vi "Error站_Core.vi"(6 "Flag in":T1, 7 "Function":T6(ring)=enum."CloseReference", 8 "error in":errorcluster, 9 "Data in":T3, 10 "Name":string, 11 "ref in":T2) -> (0 "error out":errorcluster, 2 "Data out":T3, 3 "ref out":T2, 4 "Flag out":T1)   [LabVIEW 2015]
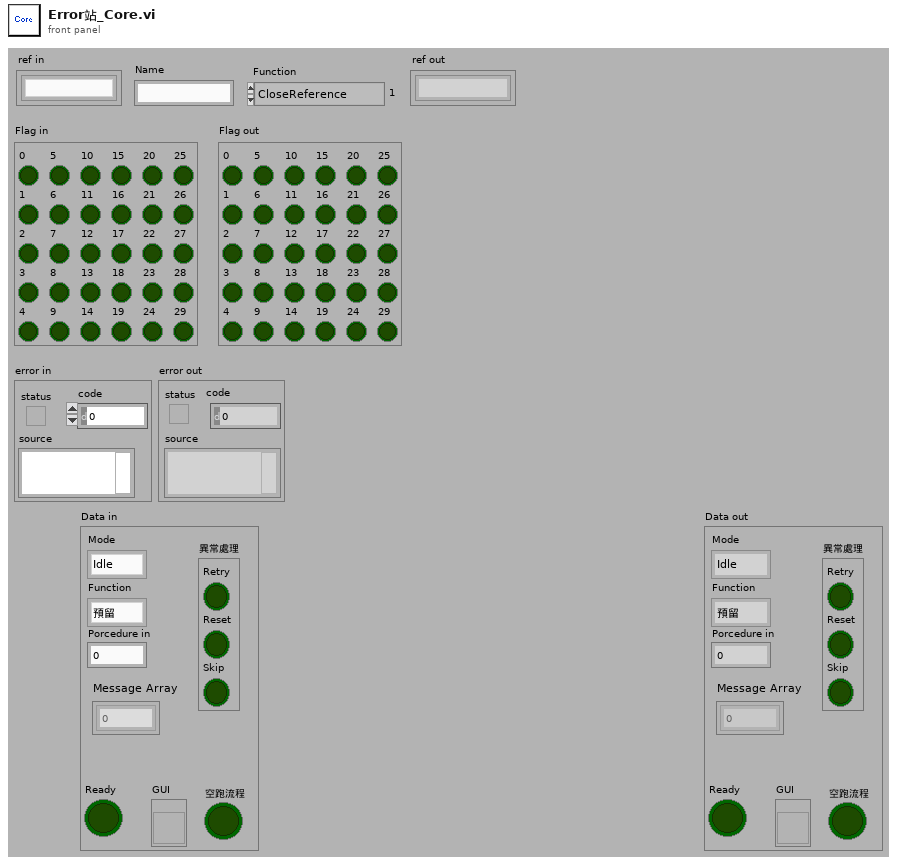
[diagram p1: front panel]
types:
  T1 = typedef "Error站_Flag.ctl" = cluster{"0":bool, "1":bool, "2":bool, "3":bool, "4":bool, "5":bool, "6":bool, "7":bool, "8":bool, "9":bool, "10":bool, "11":bool, "12":bool, "13":bool, "14":bool, "15":bool, "16":bool, "17":bool, "18":bool, "19":bool, "20":bool, "21":bool, "22":bool, "23":bool, "24":bool, "25":bool, "26":bool, "27":bool, "28":bool, "29":bool}
  T2 = typedef "Error站_ref.ctl" = refnum<k1>
  T3 = typedef "Error站_Data.ctl" = cluster{"GUI":refnum<vi>, "Ready":bool, "Mode":T4, "Function":T5, "Porcedure in":u8, "空跑流程":bool, "異常處理":cluster{"Retry":bool, "Reset":bool, "Skip":bool}, "Message Array":i32[]}
  T4 = typedef "Error站_Mode.ctl" = enum8{"Idle", "Run", "Pause", "Err"}
  T5 = typedef "Error站_Function.ctl" = enum8{"預留"}
  T6 = enum16{"OpenReference", "CloseReference", "Get Data", "Set Data", "Set Flag"}
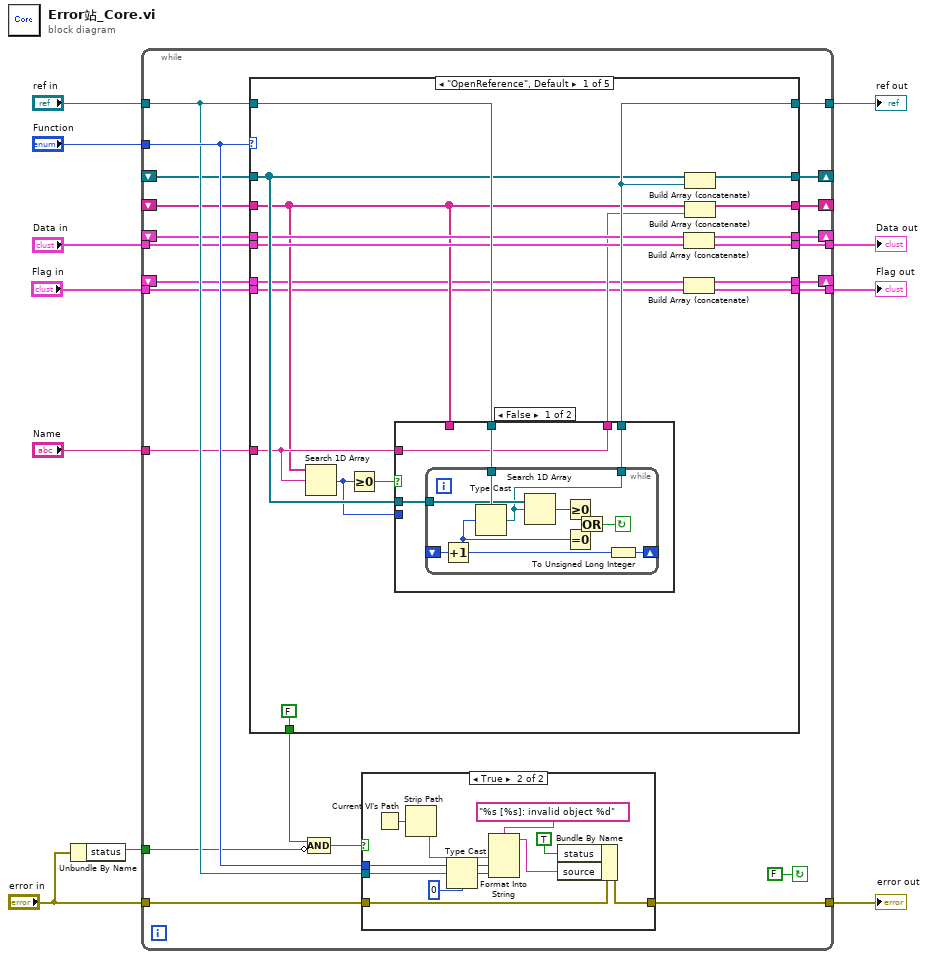
[diagram p0: block diagram]
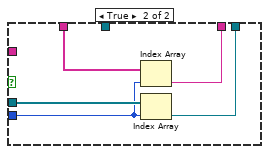
[diagram p3: hidden frame]
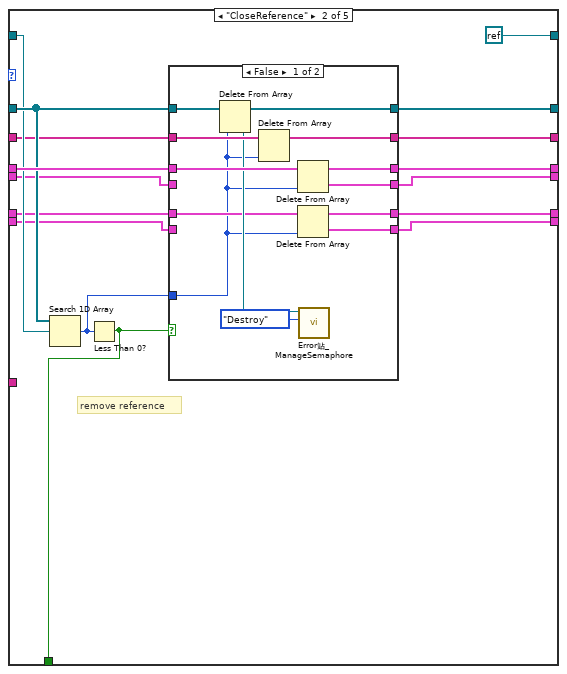
[diagram p4: hidden frame]
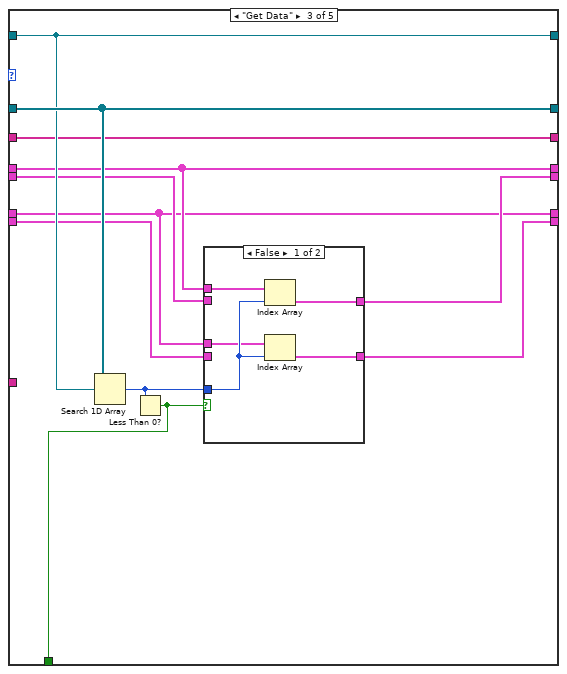
[diagram p6: hidden frame]
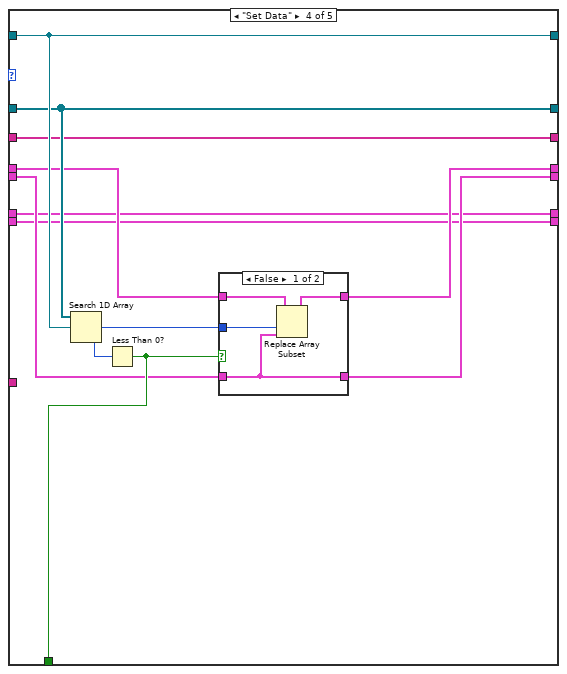
[diagram p8: hidden frame]
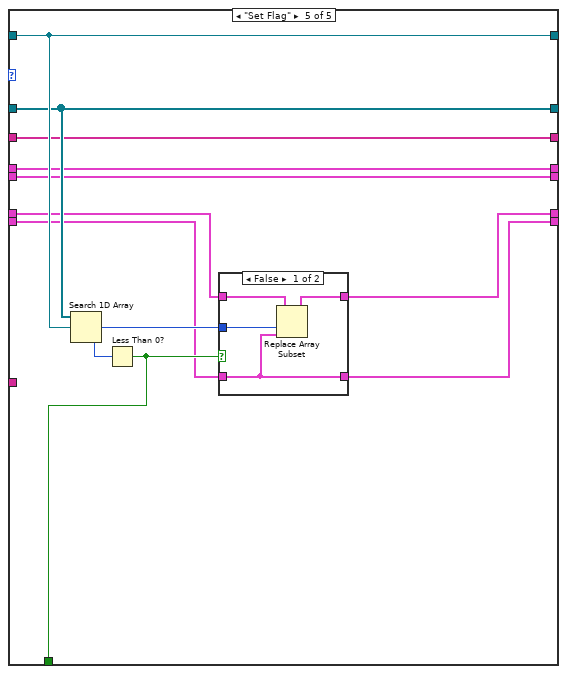
[diagram p10: hidden frame]
diagram:
  n1 = Unbundle By Name("error in") -> ("status"=w9:bool)
  n2 = while {
    tunnel: "Data in" -> [w20]
    shift-left: _ -> [w22]
    shift-right: [w21] -> _
    shift-left: _ -> [w24]
    shift-right: [w23] -> _
    tunnel: [w25] -> w3
    tunnel: w9 -> [w26]
    tunnel: [w30] -> w6
    tunnel: "error in" -> [w31]
    tunnel: "ref in" -> [w28]
    tunnel: "Function" -> [w29]
    shift-right: [w19] -> _
    shift-left: _ -> [w18]
    tunnel: "Name" -> [w17]
    tunnel: [w16] -> w4
    tunnel: "Flag in" -> [w14]
    shift-right: [w13] -> _
    shift-left: _ -> [w12]
    tunnel: [w15] -> w1
    stop <- FALSE continue-if-true
    n3 = case shown="\"OpenReference\", Default" w29 {
      tunnel: w28 -> [w62 w91 w125 w144 w161]
      tunnel: [FALSE w92 w124 w140 w159] -> w27
      tunnel: [w60 refnum<k0> refnum ("Not a Refnum Constant") w125 w144 w161] -> w25
      tunnel: w24 -> [w59 w95 w126 w143 w160]
      tunnel: [w58 w94 w126 w143 w160] -> w23
      tunnel: w22 -> [w57 w97 w123 w142 w153]
      tunnel: [w56 w96 w123 w141 w153] -> w21
      tunnel: w20 -> [w51 w87 w120 w138 w152]
      tunnel: [w55 w88 w122 w139 w158] -> w19
      tunnel: w18 -> [w50 w89 w122 w139 w158]
      tunnel: w17 -> [w52 _ _ _ _]
      tunnel: [w51 w86 w121 w137 w152] -> w16
      tunnel: w12 -> [w46 w85 w118 w136 w157]
      tunnel: [w47 w84 w118 w136 w156] -> w13
      tunnel: w14 -> [w48 w82 w117 w135 w155]
      tunnel: [w48 w83 w119 w135 w154] -> w15
      frame "OpenReference", Default {
        n4 = Search 1D Array(1D array=w50, element=w52) -> (index of element=w53:i32)  [unwired: 1 in]
        n5 = Greater Or Equal To 0?(x=w53) -> (x >= 0?=w54:bool)
        n6 = case shown="False" w54 {
          tunnel: w62 -> [w66 _]
          tunnel: [w63 w80] -> w60
          tunnel: w59 -> [w65 w81]
          tunnel: w53 -> [_ w77]
          tunnel: [w64 w78] -> w49
          tunnel: w52 -> [w64 _]
          tunnel: w50 -> [_ w79]
          frame False {
            n7 = while "Create Unique Reference" {
              tunnel: [w67] -> w63
              tunnel: w65 -> [w71]
              tunnel: w66 -> [w72]
              shift-left: _ -> [w76]
              shift-right: [w75] -> _
              stop <- w68 continue-if-true
              n8 = Increment(x=w76) -> (x+1=w74:u32)
              n9 = Type Cast(type=w72, x=w74) -> (*(type *) &x=w67:T2)
              n10 = Search 1D Array(1D array=w71, element=w67) -> (index of element=w73:i32)  [unwired: 1 in]
              n11 = Greater Or Equal To 0?(x=w73) -> (x >= 0?=w69:bool)
              n12 = Equal To 0?(x=w74) -> (x = 0?=w70:bool)
              n13 = Or(x=w69, y=w70) -> (x .or. y?=w68:bool)
              n14 = To Unsigned Long Integer(number=w74) -> (unsigned 32bit integer=w75:u32)
            }
          }
          frame True {
            n15 = Index Array(array=w79, index=w77) -> (element=w78:string)
            n16 = Index Array(array=w81, index=w77) -> (element=w80:T2)
          }
        }
        n17 = Build Array (concatenate)(w57, w51) -> (w56:T3[])
        n18 = Build Array (concatenate)(w46, w48) -> (w47:T1[])
        n19 = Build Array (concatenate)(w59, w60) -> (w58:T2[])
        n20 = Build Array (concatenate)(w50, w49) -> (w55:string[])
      }
      frame "CloseReference" {
        # "remove reference"
        n21 = Search 1D Array(1D array=w95, element=w91) -> (index of element=w93:i32)  [unwired: 1 in]
        n22 = Less Than 0?(x=w93) -> (x < 0?=w92:bool)
        n23 = case shown="False" w92 {
          tunnel: w97 -> [w106 w116]
          tunnel: [w105 w116] -> w96
          tunnel: w95 -> [w110 w115]
          tunnel: [w109 w115] -> w94
          tunnel: w93 -> [w99 _]
          tunnel: w89 -> [w108 w114]
          tunnel: [w107 w114] -> w88
          tunnel: w87 -> [_ w113]
          tunnel: [w104 w113] -> w86
          tunnel: w85 -> [w101 w112]
          tunnel: [w100 w112] -> w84
          tunnel: [w98 w111] -> w83
          tunnel: w82 -> [_ w111]
          frame False {
            n24 = Delete From Array(array=w110, index=w99) -> (deleted portion=w103:T2, array with subset deleted=w109:T2[])  [unwired: 1 in]
            n25 = Delete From Array(array=w108, index=w99) -> (array with subset deleted=w107:string[])  [unwired: 1 in, 1 out]
            n26 = Delete From Array(array=w106, index=w99) -> (deleted portion=w104:T3, array with subset deleted=w105:T3[])  [unwired: 1 in]
            n27 = Delete From Array(array=w101, index=w99) -> (deleted portion=w98:T1, array with subset deleted=w100:T1[])  [unwired: 1 in]
            n28 = call "Error站_ManageSemaphore.vi"("Method (Acquire)"=enum8{"Acquire", "Destroy"}."Destroy", "ref"=w103) -> ()  [unwired: 3 in, 3 out]
          }
          frame True {
          }
        }
      }
      frame "Get Data" {
        n29 = Search 1D Array(1D array=w126, element=w125) -> (index of element=w127:i32)  [unwired: 1 in]
        n30 = Less Than 0?(x=w127) -> (x < 0?=w124:bool)
        n31 = case shown="False" w124 {
          tunnel: w127 -> [w130 _]
          tunnel: w123 -> [w132 _]
          tunnel: [w131 w134] -> w121
          tunnel: w120 -> [_ w134]
          tunnel: w118 -> [w129 _]
          tunnel: [w128 w133] -> w119
          tunnel: w117 -> [_ w133]
          frame False {
            n32 = Index Array(array=w132, index=w130) -> (element=w131:T3)
            n33 = Index Array(array=w129, index=w130) -> (element=w128:T1)
          }
          frame True {
          }
        }
      }
      frame "Set Data" {
        n34 = Search 1D Array(1D array=w143, element=w144) -> (index of element=w145:i32)  [unwired: 1 in]
        n35 = Less Than 0?(x=w145) -> (x < 0?=w140:bool)
        n36 = case shown="False" w140 {
          tunnel: w142 -> [w149 w151]
          tunnel: [w148 w151] -> w141
          tunnel: w145 -> [w147 _]
          tunnel: w138 -> [w146 w150]
          tunnel: [w146 w150] -> w137
          frame False {
            n37 = Replace Array Subset(array=w149, new element=w146, index=w147) -> (w148:T3[])
          }
          frame True {
          }
        }
      }
      frame "Set Flag" {
        n38 = Search 1D Array(1D array=w160, element=w161) -> (index of element=w162:i32)  [unwired: 1 in]
        n39 = Less Than 0?(x=w162) -> (x < 0?=w159:bool)
        n40 = case shown="False" w159 {
          tunnel: w157 -> [w166 w168]
          tunnel: [w165 w168] -> w156
          tunnel: w162 -> [w164 _]
          tunnel: w155 -> [w163 w167]
          tunnel: [w163 w167] -> w154
          frame False {
            n41 = Replace Array Subset(array=w166, new element=w163, index=w164) -> (w165:T1[])
          }
          frame True {
          }
        }
      }
    }
    n42 = Compound Arithmetic op=AND(w27, invert w26) -> (w32:bool)
    n43 = case shown="True" w32 {
      tunnel: w29 -> [_ w43]
      tunnel: w28 -> [_ w44]
      tunnel: w31 -> [w34 w38]
      tunnel: [w34 w37] -> w30
      frame False {
      }
      frame True {
        n44 = Current VI's Path() -> (path=w42:path)
        n45 = Strip Path(path=w42) -> (name=w41:string)  [unwired: 1 out]
        n46 = Type Cast(type=u32 0 ("object"), x=w44) -> (*(type *) &x=w40:u32)
        n47 = Format Into String(format string="%s [%s]: invalid object %d", w41, w43, w40) -> (resulting string=w36:string)  [unwired: 2 in, 1 out]
        n48 = Bundle By Name(cluster=w38, "status"=TRUE, "source"=w36) -> (w37:errorcluster)
      }
    }
  }
  "error out" <- w6
  "Data out" <- w4
  "ref out" <- w3
  "Flag out" <- w1
